vi "Power Guard On Error.vi"() -> ()   [LabVIEW 2012, in "Phidget Power Guard.lvlib"]
uses:
  <instrlib>/Phidgets/Phidget Power Guard/Phidget Power Guard.lvlib
  <instrlib>/Phidgets/Phidget Power Guard/Public/PowerGuardStart.vi
  <instrlib>/Phidgets/Phidget Power Guard/Public/PowerGuardClose.vi
  <instrlib>/Phidgets/Phidget Common/Phidget Common.lvlib
panel:
  in  "Enabled":bool
  in  "Fan Mode":u32(ring)=3 items=["FAN_MODE_OFF"=1, "FAN_MODE_ON"=2, "FAN_MODE_AUTO"=3]
  in  "Over Voltage":dbl=-1.0
  out "Serial Number Return":i32
  in  "Device Info":T1={"Serial Number"=-1, "Channel"=0, "Port"=0}
  out "error out":errorcluster
  in  "stop":bool
  out "ErrorString":string
  out "ErrorCode":i32
  # "This will receive the error generated if a reading is out of range"
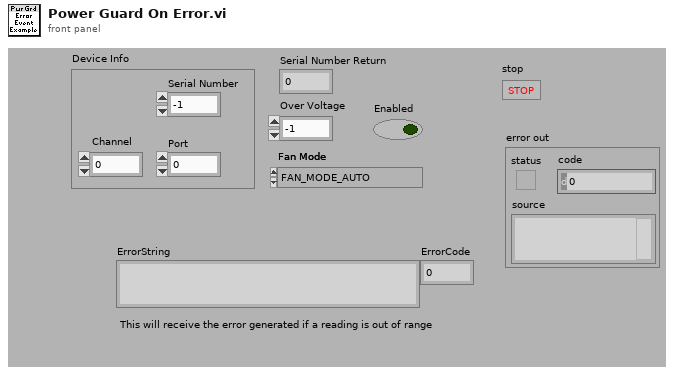
[diagram p1: front panel]
types:
  T1 = cluster{"Serial Number":i32, "Channel":i32, "Port":i32}
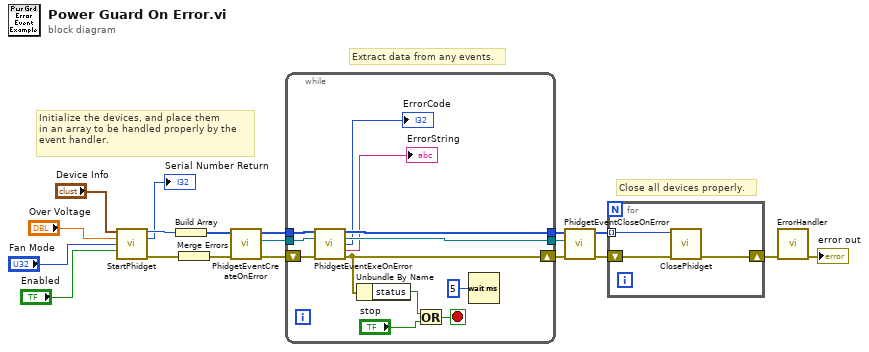
[diagram p0: block diagram]
diagram:
  # "Close all devices properly."
  # "Extract data from any events."
  # "Initialize the devices, and place them\nin an array to be handled properly by the\nevent handler."
  n1 = call-poly <instrlib>:"StartPhidget.vi"("Device Info"="Device Info", "Over Voltage"="Over Voltage", "Fan Mode"="Fan Mode", "Enabled"="Enabled") -> ("Phidget ID"=w8:u64, "Serial Number Return"=→"Serial Number Return":i32, "error out"=w4:errorcluster)  [unwired: 8 in, 1 out]
  n2 = Build Array(w8) -> (w19:u64[])
  n3 = Merge Errors(w4) -> (w10:errorcluster)
  n4 = call <instrlib>:"PhidgetEventCreateOnError.vi"("error in (no error)"=w10, "Devices In"=w19) -> ("error out"=w12:errorcluster, "Event Registration Refnum"=w17:refnum<event-registration>, "Devices Out"=w18:u64[])  [unwired: 7 in]
  n5 = while {
    tunnel: w18 -> [w31]
    tunnel: w17 -> [w27]
    tunnel: [w30] -> w14
    shift-right: [w20] -> w13
    shift-left: w12 -> [w29]
    tunnel: [w23] -> w6
    stop <- w26 stop-if-true
    n6 = call <instrlib>:"PhidgetEventExeOnError.vi"("Devices In"=w31, "Event Registration Refnum In"=w27, "error in (no error)"=w29) -> ("Devices Out"=w23:u64[], "Event Registration Refnum Out"=w30:refnum<event-registration>, "ErrorCode"=→"ErrorCode":i32, "ErrorString"=→"ErrorString":string, "error out"=w20:errorcluster)  [unwired: 5 in, 3 out]
    n7 = Unbundle By Name(w20) -> ("status"=w24:bool)
    n8 = Or(x=w24, y="stop") -> (x .or. y?=w26:bool)
    n9 = Wait (ms)(milliseconds to wait=u32 5) -> ()  [unwired: 1 out]
  }
  n10 = call <instrlib>:"PhidgetEventCloseOnError.vi"("error in (no error)"=w13, "Event Registration Refnum In"=w14, "Devices In"=w6) -> ("error out"=w9:errorcluster, "Devices Out"=w7:u64[])  [unwired: 7 in]
  n11 = for {
    tunnel: w7 -> [w32] mode=indexing
    shift-right: [w34] -> w16
    shift-left: w9 -> [w33]
    n12 = call-poly <instrlib>:"ClosePhidget.vi"("error in"=w33, "Device In"=w32) -> ("error out"=w34:errorcluster)  [unwired: 9 in]
  }
  n13 = call <instrlib>:"ErrorHandler.vi"("error in"=w16) -> ("error out"=→"error out":errorcluster)  [unwired: 9 in, 1 out]
